vi "GetNextProcessModule.vi"(8 "error in (no error)":errorcluster, 9 "data":T1, 10 "source":string, 11 "Qbus in":refnum<class "Qbus.lvclass">) -> (0 "error out":errorcluster, 3 "Qbus out":refnum<class "Qbus.lvclass">)   [LabVIEW 2017, in "DataFlow.lvlib"]
doc: "Transfers a data set to the message queue for the next process in the Dataflow Script. This VI looks up which process is next in order based on the value of the <B>source</B> input. If the <B>source</B> is the final process in Dataflow Script, this VI closes references to the data and does not send a message."
uses:
  <vilib>/addons/InsightCM/Devices/Shared/Common/DataFlow/DataFlow.lvlib
  <vilib>/addons/Qbus/Qbus.lvclass
  <vilib>/addons/InsightCM/Devices/Shared/Common/DataFlow/controls/Data.ctl
  <vilib>/addons/InsightCM/Utilities/DataAccessors/controls/wfmSGL_DVR.ctl
  <vilib>/addons/PointValueMap/controls/PointMap.ctl
  <vilib>/addons/InsightCM/Devices/Shared/Common/DataFlow/controls/Type.ctl
  <vilib>/addons/InsightCM/Devices/Shared/Common/Benchmarking/Benchmarking.lvlib
  <vilib>/addons/PointValueMap/PointValueMap.lvlib
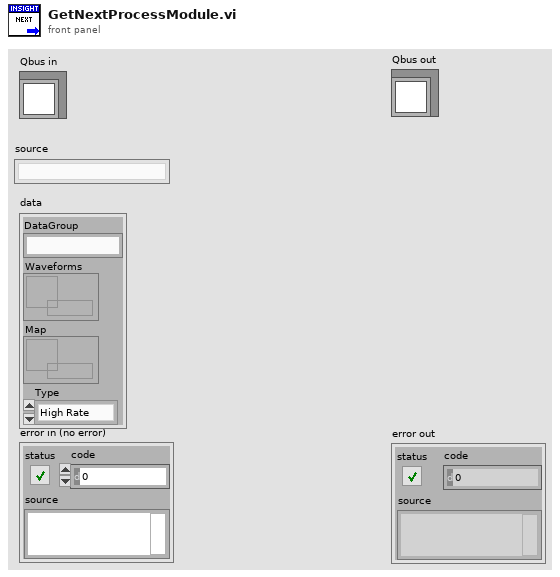
[diagram p1: front panel]
types:
  T1 = typedef "DataFlow.lvlib/Data.ctl" = cluster{"DataGroup":string, "Waveforms":T2, "Map":T3, "Type":T4}
  T2 = typedef "wfmSGL_DVR.ctl" = refnum<data-value>
  T3 = typedef "PointValueMap.lvlib/PointMap.ctl" = refnum<data-value>
  T4 = typedef "DataFlow.lvlib/Type.ctl" = enum16{"High Rate", "Low Rate", "Burst Mode"}
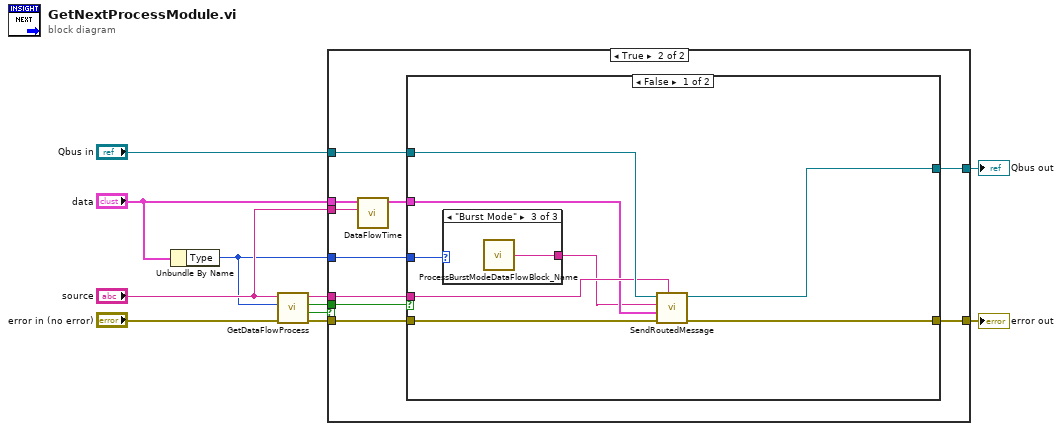
[diagram p0: block diagram]
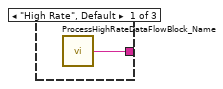
[diagram p3: hidden frame]
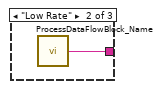
[diagram p4: hidden frame]
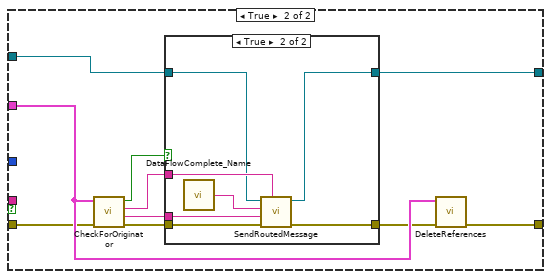
[diagram p5: hidden frame]
diagram:
  n1 = Unbundle By Name("data") -> ("Type"=w1:T4)
  n2 = call <vilib>:"GetDataFlowProcess.vi"("error in (no error)"="error in (no error)", "type"=w1, "source"="source") -> ("error out"=w10:errorcluster, "found"=w6:bool, "last block"=w4:bool, "Dataflow process"=w5:string)  [unwired: 5 in]
  n3 = case shown="True" w6 {
    tunnel: w10 -> [w12 w23]
    tunnel: [w12 w22] -> w9
    tunnel: [w13 w21] -> w8
    tunnel: "Qbus in" -> [w13 w20]
    tunnel: "data" -> [_ w18]
    tunnel: w5 -> [_ w15]
    tunnel: w4 -> [_ w19]
    tunnel: "source" -> [_ w16]
    tunnel: w1 -> [_ w14]
    frame False {
    }
    frame True {
      n4 = call <vilib>:"DataFlowTime.vi"("process"=w16, "data"=w18) -> ("data out"=w17:T1)  [unwired: 9 in]
      n5 = case shown="False" w19 {
        tunnel: w23 -> [w31 w43]
        tunnel: [w30 w42] -> w22
        tunnel: [w29 w40] -> w21
        tunnel: w20 -> [w28 w41]
        tunnel: w17 -> [w26 w44]
        tunnel: w15 -> [w27 _]
        tunnel: w14 -> [w25 _]
        frame False {
          n6 = case shown="\"Burst Mode\"" w25 {
            tunnel: [w32 w33 w34] -> w24
            frame "High Rate", Default {
              n7 = call <vilib>:"ProcessHighRateDataFlowBlock_Name.vi"() -> ("message name"=w32:string)  [unwired: 5 in]
            }
            frame "Low Rate" {
              n8 = call <vilib>:"ProcessDataFlowBlock_Name.vi"() -> ("message name"=w33:string)  [unwired: 5 in]
            }
            frame "Burst Mode" {
              n9 = call <vilib>:"ProcessBurstModeDataFlowBlock_Name.vi"() -> ("message name"=w34:string)  [unwired: 5 in]
            }
          }
          n10 = call <vilib>:"SendRoutedMessage.vi"("listener process"=w27, "error in (no error)"=w31, "message value"=w26, "message name"=w24, "Qbus in"=w28) -> ("error in (no error)"=w30:errorcluster, "Qbus out"=w29:refnum<class "Qbus.lvclass">)  [unwired: 5 in]
        }
        frame True {
          n11 = call <vilib>:"CheckForOriginator.vi"("error in (no error)"=w43, "data in"=w44) -> ("error out"=w36:errorcluster, "group"=w37:string, "originator"=w38:string, "found"=w39:bool)  [unwired: 6 in]
          n12 = case shown="True" w39 {
            tunnel: w36 -> [w45 w52]
            tunnel: [w45 w51] -> w35
            tunnel: w38 -> [_ w53]
            tunnel: w41 -> [w46 w50]
            tunnel: [w46 w49] -> w40
            tunnel: w37 -> [_ w47]
            frame False {
            }
            frame True {
              n13 = call <vilib>:"DataFlowComplete_Name.vi"() -> ("message name"=w48:string)  [unwired: 5 in]
              n14 = call <vilib>:"SendRoutedMessage.vi"("listener process"=w53, "error in (no error)"=w52, "message value"=w47, "message name"=w48, "Qbus in"=w50) -> ("error in (no error)"=w51:errorcluster, "Qbus out"=w49:refnum<class "Qbus.lvclass">)  [unwired: 5 in]
            }
          }
          n15 = call <vilib>:"DeleteReferences.vi"("error in (no error)"=w35, "data in"=w44) -> ("error out"=w42:errorcluster)  [unwired: 9 in]
        }
      }
    }
  }
  "error out" <- w9
  "Qbus out" <- w8
